vi "FlujoDeDatos.vi"() -> ()   [LabVIEW 2022 SP3]
panel:
  out "Promedio":dbl
  in  "N2":dbl
  in  "N1":dbl
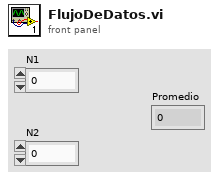
[diagram p1: front panel]
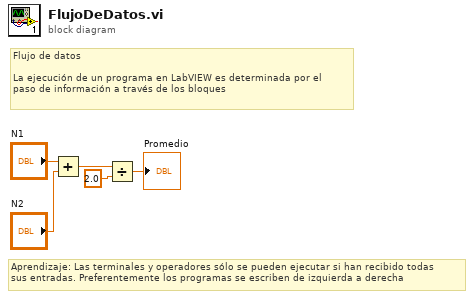
[diagram p0: block diagram]
diagram:
  # "Aprendizaje: Las terminales y operadores sólo se pueden ejecutar si han recibido todas\nsus entradas. Preferentemente los programas se escriben de izquierda a derecha"
  # "Flujo de datos\n\nLa ejecución de un programa en LabVIEW es determinada por el \npaso de información a través de los bloques"
  n1 = Add(x="N1", y="N2") -> (x+y=w3:dbl)
  n2 = Divide(x=w3, y=2.0) -> (x/y=→"Promedio":dbl)
